vi "Reduce maxMFC 2 MFC count index for Pump index.vi"(11 "MFC idx":i32) -> (0 "Pump":bool, 1 "Pump Idx":i32, 3 "AutoLin MFC":i32)   [LabVIEW 2020, in "Linearisierung v2.lvlib" / "Gasteiler.lvlib" / "HovaCAL_Interface.lvlib" / "Helper.lvlib"]
uses:
  Helper.lvlib
  Kommunikation/Aktion_FGV_HovaCAL_Interface_GetData.ctl
  Kommunikation/Kommunikation.lvlib
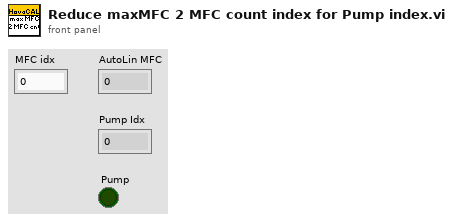
[diagram p1: front panel]
types:
  T1 = typedef "Linearisierung v2.lvlib/Gasteiler.lvlib/HovaCAL_Interface.lvlib/Kommunikation.lvlib/Aktion_FGV_HovaCAL_Interface_GetData.ctl" = enum16{"lesen", "SystemInfo", "MFC Info", "actual Values", "Limits", "first contact"}
  T2 = typedef "Linearisierung v2.lvlib/Gasteiler.lvlib/HovaCAL_Interface.lvlib/Controls.lvlib/Info Cluster.ctl" = cluster{"device":string, "version":string, "number of mfc":i32, "number of pumps":i32, "number of temp controllers":i32, "number of mfs":i32, "number of balances":i32}
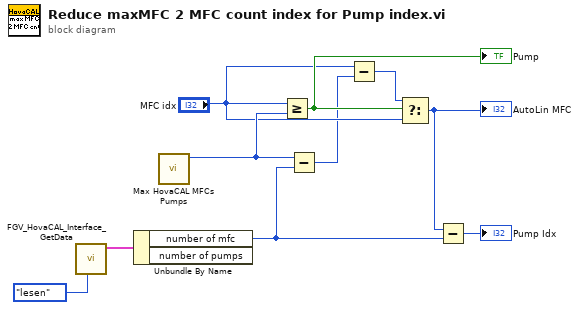
[diagram p0: block diagram]
diagram:
  n1 = call "FGV_HovaCAL_Interface_GetData.vi"("Aktion"=Aktion_FGV_HovaCAL_Interface_GetData."lesen") -> ("System Cluster out"=w9:T2)  [unwired: 6 in, 4 out]
  n2 = Unbundle By Name(w9) -> ("number of mfc"=w2:i32)  [unwired: 1 out]
  n3 = call "Max HovaCAL MFCs Pumps.vi"() -> ("max MFCs"=w8:i32)  [unwired: 10 in, 1 out]
  n4 = Greater Or Equal?(x="MFC idx", y=w8) -> (x >= y?=w7:bool)
  "Pump" <- w7
  n5 = Subtract(x=w8, y=w2) -> (x-y=w5:i32)
  n6 = Subtract(x="MFC idx", y=w5) -> (x-y=w4:i32)
  n7 = Select(t=w4, s=w7, f="MFC idx") -> (s? t:f=w3:i32)
  "AutoLin MFC" <- w3
  n8 = Subtract(x=w3, y=w2) -> (x-y=→"Pump Idx":i32)
